vi "SL_ReadData.vi"(11 "Property":string) -> (1 "type":string, 2 "value":string)   [LabVIEW 2020]
panel:
  out "Value Read":string
  out "Number Read":dbl
  out "Comm":T1
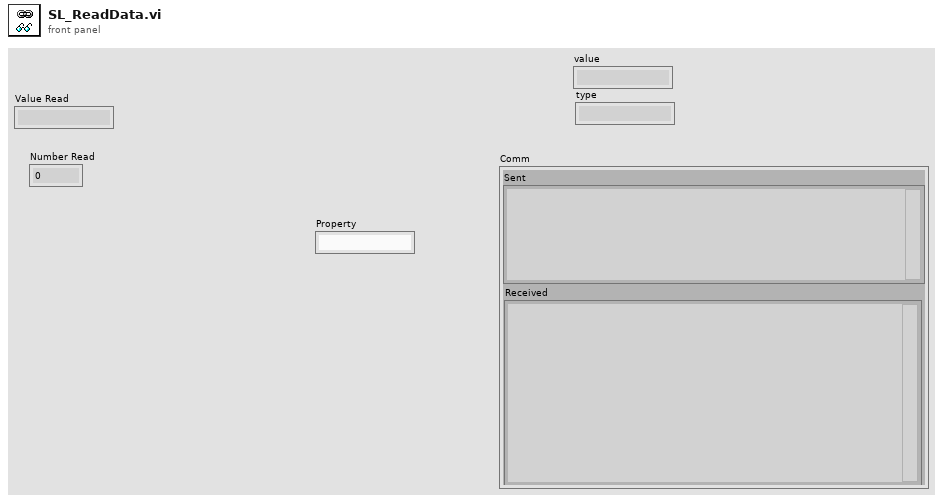
[diagram p1: front panel]
types:
  T1 = cluster{"url":string, "sent headers":string, "sent body":string, "headers":string, "body":string, "Sent":string, "Received":string}
  T2 = enum16{"GET", "PUT", "POST", "MultiPOST", "DELETE"}
  T3 = cluster{"current":cluster{"timestamp":string, "value":cluster{"type":string, "value":string}}}
  T4 = cluster{"Name":string, "BaseURL":string, "AppKey":string, "Headers":string[], "Timeout":i32}
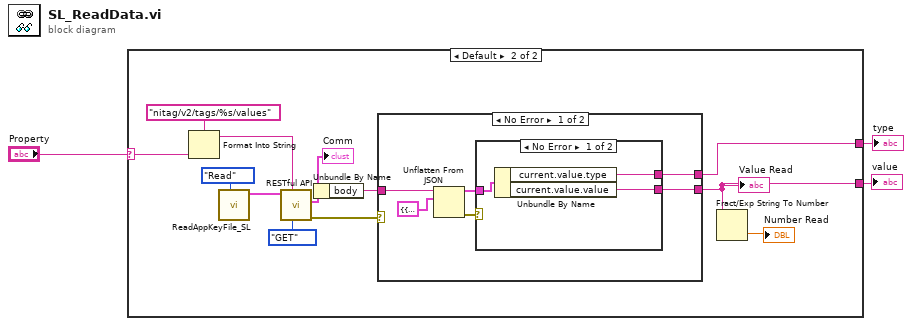
[diagram p0: block diagram]
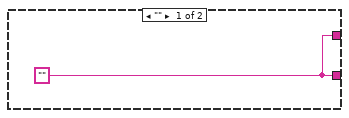
[diagram p2: hidden frame]
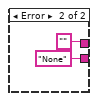
[diagram p3: hidden frame]
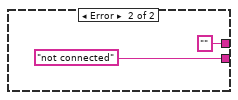
[diagram p4: hidden frame]
diagram:
  n1 = case shown="Default" "Property" {
    selector: "Property" -> [_ w11]
    tunnel: [w4 w6] -> w3
    tunnel: [w4 w5] -> w2
    frame "" {
      w4 = "" ("body")
    }
    frame Default {
      n2 = Format Into String(format string="nitag/v2/tags/%s/values" ("url"), w11) -> (resulting string=w10:string)  [unwired: 2 in, 1 out]
      n3 = call "ReadAppKeyFile_SL.vi"("Task"=enum16{"Read", "Write"}."Read") -> ("Device Out"=w16:T4)  [unwired: 8 in, 2 out]
      n4 = call "RESTful API.vi"("Method"=T2."GET", "url"=w10, "Device In"=w16) -> ("error out"=w7:errorcluster, "Comm"=w9:T1)  [unwired: 6 in, 1 out]
      "Comm" <- w9
      n5 = Unbundle By Name(w9) -> ("body"=w8:string)
      n6 = case shown="No Error" w7 {
        tunnel: [w18 "not connected" ("value")] -> w6
        tunnel: w8 -> [w19 _]
        tunnel: [w17 "" ("type")] -> w5
        frame No Error {
          n7 = Unflatten From JSON(JSON string=w19, type and defaults=T3 {"current"={"timestamp"="", "value"={"type"="", "value"=""}}}) -> (value=w20:T3, error out=w21:errorcluster)  [unwired: 5 in]
          n8 = case shown="No Error" w21 {
            tunnel: w20 -> [w25 _]
            tunnel: [w24 "None" ("value")] -> w18
            tunnel: [w23 "" ("type")] -> w17
            frame No Error {
              n9 = Unbundle By Name(w25) -> ("current.value.type"=w23:string, "current.value.value"=w24:string)
            }
            frame Error {
            }
          }
        }
        frame Error {
        }
      }
      "Value Read" <- w6
      n10 = Fract/Exp String To Number(string=w6) -> (number=→"Number Read":dbl)  [unwired: 3 in, 1 out]
    }
  }
  "value" <- w3
  "type" <- w2
